vi "XPath Queries for Prof Watts.vi"() -> ()   [LabVIEW 2013, in "XML.lvlib"]
uses:
  XML.lvlib
  <resource>/objmgr/DOMUserDefRef.rc
panel:
  in  "Original Document":string="<?xml version=\"1.0\" encoding=\"UTF-8\"?>\n<office:document-content xmlns:office=\"urn:oasis:names:tc:opendocument:xmlns:office:1.0\" xmlns:style=\"urn:oasis:names:tc:opendocument:xmlns:style:1.0\" xmlns:text=\"urn:oasis:names:tc:opendocument:xmlns:text:1.0\" xmlns:table=\"urn:oasis:names:tc:opendocument:xmlns:table:1.0\" xmlns:draw=\"urn:oasis:names:tc:opendocument:xmlns:drawing:1.0\" xmlns:fo=\"urn:oasis:names:tc:opendocument:xmlns:xsl-fo-compatible:1.0\" xmlns:xlink=\"http://www.w3.org/1999/xlink\" xmlns:dc=\"http://purl.org/dc/elements/1.1/\" xmlns:meta=\"urn:oasis:names:tc:opendocument:xmlns:meta:1.0\" xmlns:number=\"urn:oasis:names:tc:opendocument:xmlns:datastyle:1.0\" xmlns:presentation=\"urn:oasis:names:tc:opendocument:xmlns:presentation:1.0\" xmlns:svg=\"urn:oasis:names:tc:opendocument:xmlns:svg-compatible:1.0\" xmlns:chart=\"urn:oasis:names:tc:opendocument:xmlns:chart:1.0\" xmlns:dr3d=\"urn:oasis:names:tc:opendocument:xmlns:dr3d:1.0\" xmlns:math=\"http://www.w3.org/1998/Math/MathML\" xmlns:form=\"urn:oasis:names:tc:opendocument:xmlns:form:1.0\" xmlns:script=\"urn:oasis:names:tc:opendocument:xmlns:script:1.0\" xmlns:ooo=\"http://openoffice.org/2004/office\" xmlns:ooow=\"http://openoffice.org/2004/writer\" xmlns:oooc=\"http://openoffice.org/2004/calc\" xmlns:dom=\"http://www.w3.org/2001/xml-events\" xmlns:xforms=\"http://www.w3.org/2002/xforms\" xmlns:xsd=\"http://www.w3.org/2001/XMLSchema\" xmlns:xsi=\"http://www.w3.org/2001/XMLSchema-instance\" xmlns:rpt=\"http://openoffice.org/2005/report\" xmlns:of=\"urn:oasis:names:tc:opendocument:xmlns:of:1.2\" xmlns:xhtml=\"http://www.w3.org/1999/xhtml\" xmlns:grddl=\"http://www.w3.org/2003/g/data-view#\" xmlns:tableooo=\"http://openoffice.org/2009/table\" xmlns:drawooo=\"http://openoffice.org/2010/draw\" xmlns:calcext=\"urn:org:documentfoundation:names:experimental:calc:xmlns:calcext:1.0\" xmlns:loext=\"urn:org:documentfoundation:names:experimental:office:xmlns:loext:1.0\" xmlns:field=\"urn:openoffice:names:experimental:ooo-ms-interop:xmlns:field:1.0\" xmlns:formx=\"urn:openoffice:names:experimental:ooxml-odf-interop:xmlns:form:1.0\" xmlns:css3t=\"http://www.w3.org/TR/css3-text/\" office:version=\"1.2\">\n\t<office:scripts/>\n\t<office:font-face-decls>\n\t\t<style:font-face style:name=\"Arial\" svg:font-family=\"Arial\" style:font-family-generic=\"swiss\" style:font-pitch=\"variable\"/>\n\t\t<style:font-face style:name=\"Mangal\" svg:font-family=\"Mangal\" style:font-family-generic=\"system\" style:font-pitch=\"variable\"/>\n\t\t<style:font-face style:name=\"Microsoft YaHei\" svg:font-family=\"&apos;Microsoft YaHei&apos;\" style:font-family-generic=\"system\" style:font-pitch=\"variable\"/>\n\t\t<style:font-face style:name=\"Segoe UI\" svg:font-family=\"&apos;Segoe UI&apos;\" style:font-family-generic=\"system\" style:font-pitch=\"variable\"/>\n\t\t<style:font-face style:name=\"Tahoma\" svg:font-family=\"Tahoma\" style:font-family-generic=\"system\" style:font-pitch=\"variable\"/>\n\t</office:font-face-decls>\n\t<office:automatic-styles>\n\t\t<style:style style:name=\"co1\" style:family=\"table-column\">\n\t\t\t<style:table-column-properties fo:break-before=\"auto\" style:column-width=\"2.258cm\"/>\n\t\t</style:style>\n\t\t<style:style style:name=\"co2\" style:family=\"table-column\">\n\t\t\t<style:table-column-properties fo:break-before=\"auto\" style:column-width=\"5.999cm\"/>\n\t\t</style:style>\n\t\t<style:style style:name=\"ro1\" style:family=\"table-row\">\n\t\t\t<style:table-row-properties style:row-height=\"0.453cm\" fo:break-before=\"auto\" style:use-optimal-row-height=\"true\"/>\n\t\t</style:style>\n\t\t<style:style style:name=\"ro2\" style:family=\"table-row\">\n\t\t\t<style:table-row-properties style:row-height=\"0.473cm\" fo:break-before=\"auto\" style:use-optimal-row-height=\"true\"/>\n\t\t</style:style>\n\t\t<style:style style:name=\"ta1\" style:family=\"table\" style:master-page-name=\"Default\">\n\t\t\t<style:table-properties table:display=\"true\" style:writing-mode=\"lr-tb\"/>\n\t\t</style:style>\n\t</office:automatic-styles>\n\t<office:body>\n\t\t<office:spreadsheet>\n\t\t\t<table:table table:name=\"Sheet1\" table:style-name=\"ta1\">\n\t\t\t\t<table:table-column table:style-name=\"co1\" table:default-cell-style-name=\"Default\"/>\n\t\t\t\t<table:table-column table:style-name=\"co2\" table:default-cell-style-name=\"Default\"/>\n\t\t\t\t<table:table-column table:style-name=\"co1\" table:number-columns-repeated=\"11\" table:default-cell-style-name=\"Default\"/>\n\t\t\t\t<table:table-row table:style-name=\"ro1\">\n\t\t\t\t\t<table:table-cell office:value-type=\"string\" calcext:value-type=\"string\">\n\t\t\t\t\t\t<text:p>Title1</text:p>\n\t\t\t\t\t</table:table-cell>\n\t\t\t\t\t<table:table-cell table:number-columns-repeated=\"12\"/>\n\t\t\t\t</table:table-row>\n\t\t\t\t<table:table-row table:style-name=\"ro2\">\n\t\t\t\t\t<table:table-cell/>\n\t\t\t\t\t<table:table-cell office:value-type=\"string\" calcext:value-type=\"string\">\n\t\t\t\t\t\t<text:p>aaaaaaaaaaaaaaaaaaaaa</text:p>\n\t\t\t\t\t</table:table-cell>\n\t\t\t\t\t<table:table-cell table:number-columns-repeated=\"5\"/>\n\t\t\t\t\t<table:table-cell office:value-type=\"string\" calcext:value-type=\"string\">\n\t\t\t\t\t\t<text:p>H2</text:p>\n\t\t\t\t\t</table:table-cell>\n\t\t\t\t\t<table:table-cell table:number-columns-repeated=\"5\"/>\n\t\t\t\t</table:table-row>\n\t\t\t\t<table:table-row table:style-name=\"ro2\">\n\t\t\t\t\t<table:table-cell/>\n\t\t\t\t\t<table:table-cell office:value-type=\"string\" calcext:value-type=\"string\">\n\t\t\t\t\t\t<text:p>bbbbbbbbbbbbbbbbbbbbb</text:p>\n\t\t\t\t\t</table:table-cell>\n\t\t\t\t\t<table:table-cell table:number-columns-repeated=\"11\"/>\n\t\t\t\t</table:table-row>\n\t\t\t\t<table:table-row table:style-name=\"ro2\">\n\t\t\t\t\t<table:table-cell/>\n\t\t\t\t\t<table:table-cell office:value-type=\"string\" calcext:value-type=\"string\">\n\t\t\t\t\t\t<text:p>ccccccccccccccccccccc</text:p>\n\t\t\t\t\t</table:table-cell>\n\t\t\t\t\t<table:table-cell table:number-columns-repeated=\"11\"/>\n\t\t\t\t</table:table-row>\n\t\t\t\t<table:table-row table:style-name=\"ro2\">\n\t\t\t\t\t<table:table-cell/>\n\t\t\t\t\t<table:table-cell office:value-type=\"string\" calcext:value-type=\"string\">\n\t\t\t\t\t\t<text:p>ddddddddddddddddddddd</text:p>\n\t\t\t\t\t</table:table-cell>\n\t\t\t\t\t<table:table-cell table:number-columns-repeated=\"11\"/>\n\t\t\t\t</table:table-row>\n\t\t\t\t<table:table-row table:style-name=\"ro1\">\n\t\t\t\t\t<table:table-cell office:value-type=\"string\" calcext:value-type=\"string\">\n\t\t\t\t\t\t<text:p>Title2</text:p>\n\t\t\t\t\t</table:table-cell>\n\t\t\t\t\t<table:table-cell table:number-columns-repeated=\"12\"/>\n\t\t\t\t</table:table-row>\n\t\t\t\t<table:table-row table:style-name=\"ro2\">\n\t\t\t\t\t<table:table-cell/>\n\t\t\t\t\t<table:table-cell office:value-type=\"string\" calcext:value-type=\"string\">\n\t\t\t\t\t\t<text:p>eeeeeeeeeeeeeeeeeeeee</text:p>\n\t\t\t\t\t</table:table-cell>\n\t\t\t\t\t<table:table-cell table:number-columns-repeated=\"11\"/>\n\t\t\t\t</table:table-row>\n\t\t\t\t<table:table-row table:style-name=\"ro2\">\n\t\t\t\t\t<table:table-cell/>\n\t\t\t\t\t<table:table-cell office:value-type=\"string\" calcext:value-type=\"string\">\n\t\t\t\t\t\t<text:p>ffffffffffffffffffffffffffffffffffffffff</text:p>\n\t\t\t\t\t</table:table-cell>\n\t\t\t\t\t<table:table-cell table:number-columns-repeated=\"11\"/>\n\t\t\t\t</table:table-row>\n\t\t\t\t<table:table-row table:style-name=\"ro1\">\n\t\t\t\t\t<table:table-cell/>\n\t\t\t\t\t<table:table-cell office:value-type=\"string\" calcext:value-type=\"string\">\n\t\t\t\t\t\t<text:p>ggggggggggggggggggggg</text:p>\n\t\t\t\t\t</table:table-cell>\n\t\t\t\t\t<table:table-cell table:number-columns-repeated=\"11\"/>\n\t\t\t\t</table:table-row>\n\t\t\t\t<table:table-row table:style-name=\"ro1\" table:number-rows-repeated=\"5\">\n\t\t\t\t\t<table:table-cell table:number-columns-repeated=\"13\"/>\n\t\t\t\t</table:table-row>\n\t\t\t\t<table:table-row table:style-name=\"ro1\">\n\t\t\t\t\t<table:table-cell table:number-columns-repeated=\"4\"/>\n\t\t\t\t\t<table:table-cell office:value-type=\"string\" calcext:value-type=\"string\">\n\t\t\t\t\t\t<text:p>E16</text:p>\n\t\t\t\t\t</table:table-cell>\n\t\t\t\t\t<table:table-cell table:number-columns-repeated=\"8\"/>\n\t\t\t\t</table:table-row>\n\t\t\t\t<table:table-row table:style-name=\"ro1\" table:number-rows-repeated=\"10\">\n\t\t\t\t\t<table:table-cell table:number-columns-repeated=\"13\"/>\n\t\t\t\t</table:table-row>\n\t\t\t\t<table:table-row table:style-name=\"ro1\">\n\t\t\t\t\t<table:table-cell table:number-columns-repeated=\"12\"/>\n\t\t\t\t\t<table:table-cell office:value-type=\"string\" calcext:value-type=\"string\">\n\t\t\t\t\t\t<text:p>M26</text:p>\n\t\t\t\t\t</table:table-cell>\n\t\t\t\t</table:table-row>\n\t\t\t</table:table>\n\t\t\t<table:named-expressions/>\n\t\t</office:spreadsheet>\n\t</office:body>\n</office:document-content>"
  in  "XPath Query":string="/office:document-content/office:body/office:spreadsheet/table:table/table:table-row"
  out "Results":string[](array[string])
  out "error out":errorcluster
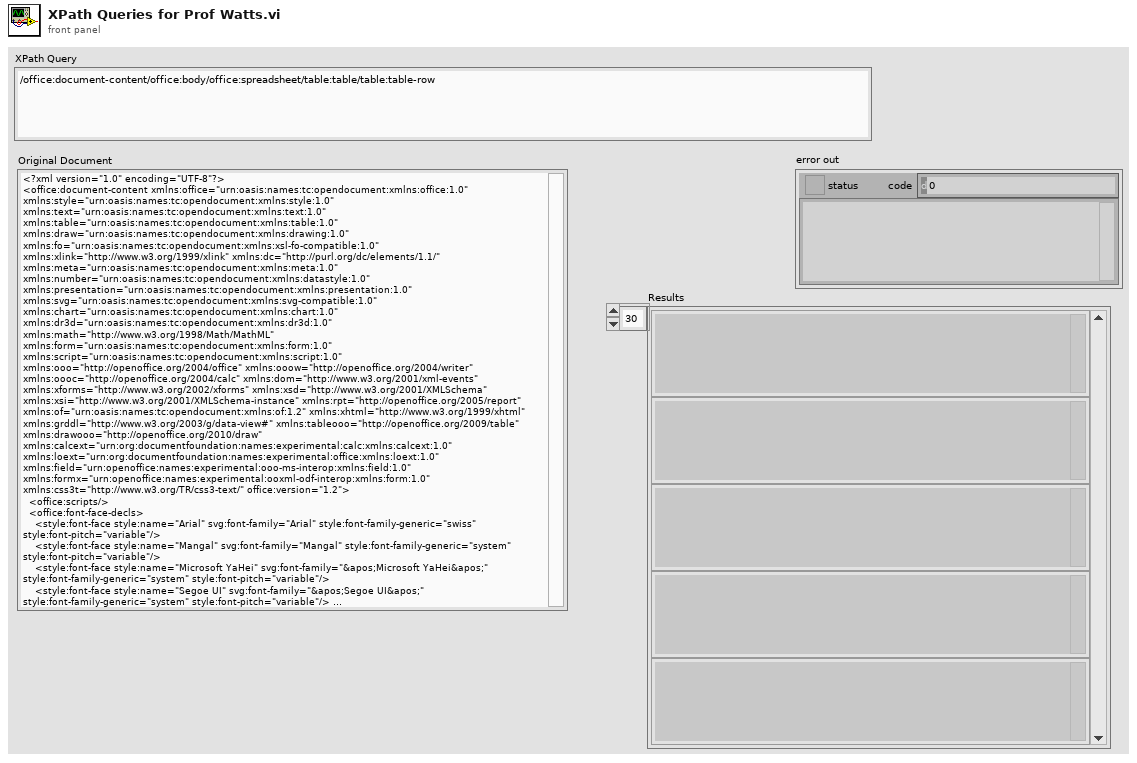
[diagram p1: front panel]
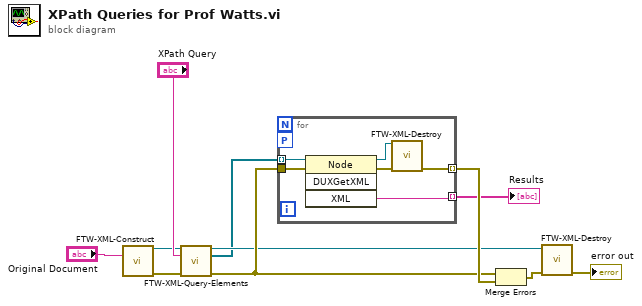
[diagram p0: block diagram]
diagram:
  n1 = call "FTW-XML-Construct.vi"("XML String"="Original Document") -> ("XML Document"=w7:refnum<k20>, "error out"=w10:errorcluster)  [unwired: 13 in]
  n2 = call "FTW-XML-Query-Elements.vi"("XML Node"=w7, "XPath Query"="XPath Query", "error in"=w10) -> ("XML Node out"=w3:refnum<k20>, "Matching Nodes"=w2:refnum<k20>[], "error out"=w5:errorcluster)  [unwired: 9 in, 1 out]
  n3 = for {
    tunnel: w2 -> [w16] mode=indexing
    workers-P: _ -> [_]
    tunnel: w5 -> [w15]
    tunnel: [w17] -> w6 mode=indexing
    tunnel: [w14] -> w1 mode=indexing
    n4 = invoke class="Node" method="DUXGetXML"(reference=w16, error in=w15) -> (reference out=w12:refnum<k20>, error out=w13:errorcluster, "XML"=w14:string)  [unwired: 2 in, 1 out]
    n5 = call "FTW-XML-Destroy.vi"("XML Node"=w12, "error in"=w13) -> ("error out"=w17:errorcluster)  [unwired: 13 in]
  }
  "Results" <- w1
  n6 = Merge Errors(w5, w6) -> (w4:errorcluster)
  n7 = call "FTW-XML-Destroy.vi"("XML Node"=w3, "error in"=w4) -> ("error out"=→"error out":errorcluster)  [unwired: 13 in]
